vi "Read password.vi"(8 "error in (no error)":errorcluster, 11 "SetEngineerAccessMode in":refnum<class "SetEngineerAccessMode.lvclass">) -> (0 "error out":errorcluster, 2 "password":string, 3 "SetEngineerAccessMode out":refnum<class "SetEngineerAccessMode.lvclass">)   [LabVIEW 2022 SP3, in "TCSDataDefinitions.lvlib" / "TCSCommand.lvlib" / "SetAccessMode.lvlib" / "SetEngineerAccessMode.lvclass"]
uses:
  SetEngineerAccessMode.lvclass
  SetEngineerAccessMode.lvclass/SetEngineerAccessMode.ctl
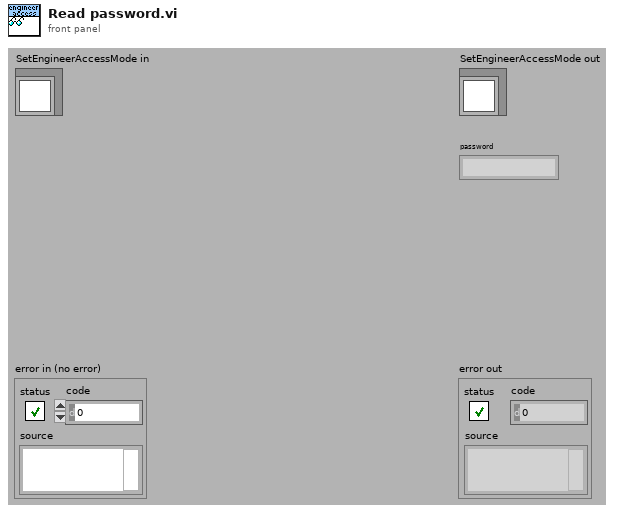
[diagram p1: front panel]
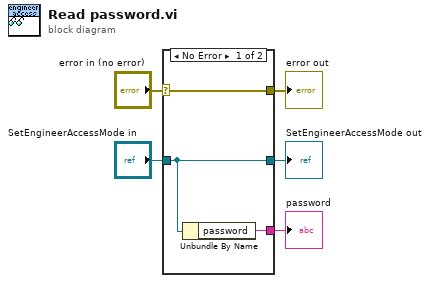
[diagram p0: block diagram]
diagram:
  n1 = case shown="No Error" "error in (no error)" {
    selector: "error in (no error)" -> [w8 w9]
    tunnel: [w8 w9] -> w4
    tunnel: [w7 w10] -> w2
    tunnel: "SetEngineerAccessMode in" -> [w7 w10]
    tunnel: [w6 _] -> w1
    frame No Error {
      n2 = Unbundle By Name(w7) -> ("password"=w6:string)
    }
    frame Error {
    }
  }
  "error out" <- w4
  "SetEngineerAccessMode out" <- w2
  "password" <- w1
